vi "Initialize.vi"(8 "error in":errorcluster, 9 "Application Directory":path, 10 "Device":string, 11 "DIG_IO in":refnum<class "DIG_IO.lvclass">) -> (0 "error out":errorcluster, 3 "DIG_IO out":refnum<class "DIG_IO.lvclass">)   [LabVIEW 2019, in "DIG_IO.lvlib" / "DIG_IO.lvclass"]
doc: "This routine instantiates a Digital IO Driver by reading the resource address, number of digital inputs and number of digital outputs controlled by the digital IO card. It then initializes two 1d boolean arrays: \nDigital In\nDigital Out\n\nThese arrays will hold the state information for the Digital Inputs and Outputs respectively."
uses:
  Library/DIG_IO.lvclass
  builds/Instruments/Instruments.lvlibp/Library/Instruments.lvclass
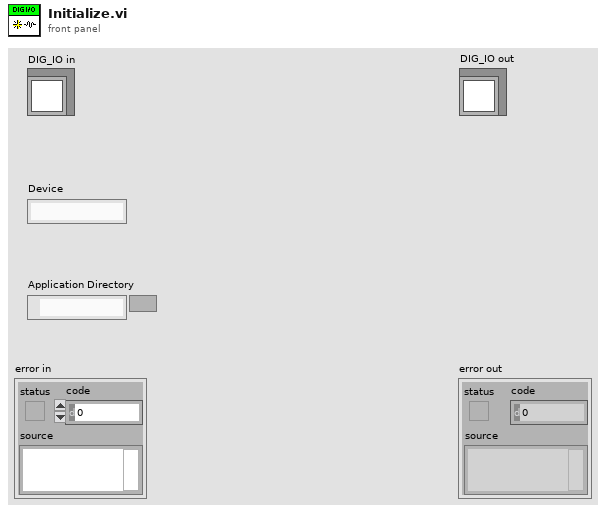
[diagram p1: front panel]
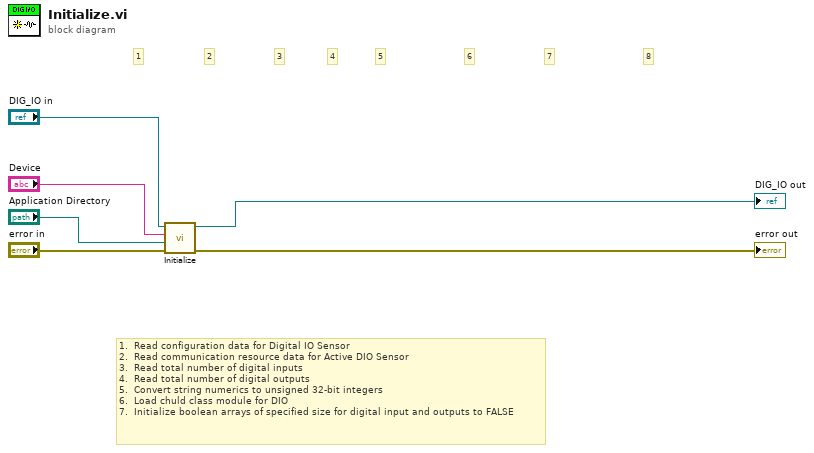
[diagram p0: block diagram]
diagram:
  # "1.  Read configuration data for Digital IO Sensor\n2.  Read communication resource data for Active DIO Sensor\n3.  Read total number of digital inputs\n4.  Read total number of digital outputs\n5.  Convert string numerics to unsigned 32-bit integers\n6.  Load chuld class module for DIO\n7.  Initialize boolean arrays of specified size for digital input and outputs to FALSE"
  # "8"
  # "7"
  # "6"
  # "5"
  # "4"
  # "3"
  # "2"
  # "1"
  n1 = call-parent "Initialize.vi"("error in"="error in", "Path"="Application Directory", "Device"="Device", "Instruments in"="DIG_IO in") -> ("error out"=→"error out":errorcluster, "Instruments out"=→"DIG_IO out":refnum<class "DIG_IO.lvclass">)  [unwired: 6 in]
